vi "Turret_Begin.vi"   [LabVIEW 2019]
uses:
  Turret_Cluster.ctl
  Turret_States.ctl
  Globals/Turret_Globals.vi
types:
  T1 = typedef "Turret_Cluster.ctl" = cluster{"Auto-Target?":bool, "Control_State":T2, "Turret_Spin_Speed":dbl, "Turret_Spin_Speed_Control?":bool, "Step":dbl, "Parameter_1":dbl, "Parameter_2":dbl, "Parameter_3":dbl, "Auto_Notifier":refnum<notifier>, "GoToZero?":bool}
  T2 = typedef "Turret_States.ctl" = enum16{"Manual_Percent_Voltage", "Manual_Speed_Control", "Auto-Target", "Command_TurnToPosition", "Command_Auto_Target", "GoToZero"}
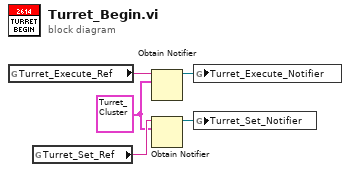
[diagram p0: block diagram]
diagram:
  w3 = T1 {"Auto-Target?"=FALSE, "Control_State"=enum."Manual_Percent_Voltage", "Turret_Spin_Speed"=0.0, "Turret_Spin_Speed_Control?"=FALSE, "Step"=0.0, "Parameter_1"=0.0, "Parameter_2"=0.0, "Parameter_3"=0.0, "Auto_Notifier"=refnum, "GoToZero?"=FALSE} ("Turret_Cluster")
  n1 = global read "Turret_Globals.vi" "Turret_Execute_Ref"() -> (w5:string)
  n2 = global read "Turret_Globals.vi" "Turret_Set_Ref"() -> (w4:string)
  n3 = Obtain Notifier(name (unnamed)=w5, notification data type=w3) -> (notifier out=w2:refnum<notifier>)  [unwired: 2 in, 2 out]
  n4 = Obtain Notifier(name (unnamed)=w4, notification data type=w3) -> (notifier out=w1:refnum<notifier>)  [unwired: 2 in, 2 out]
  n5 = global write "Turret_Globals.vi" "Turret_Execute_Notifier"(w2) -> ()
  n6 = global write "Turret_Globals.vi" "Turret_Set_Notifier"(w1) -> ()
